vi "CCSelectDICOMitemTags.vi"() -> ()   [LabVIEW 2013, in "ClearCanvasLibrary.lvlib"]
uses:
  ClearCanvasLibrary.lvlib
  main.lvlib
  C:/Users/Simon/SkyDrive/LabView/2013/DM2020/DICOM/ClearCanvasNewBuild/ClearCanvas.Dicom.dll
  ClearCanvasNewBuild/ClearCanvas.Dicom.dll
panel:
  out "Item Symbols":i32[](array[numeric])
  in  "Listbox":i32[](listbox)
  out "error out":errorcluster
  in  "error in (no error)":errorcluster
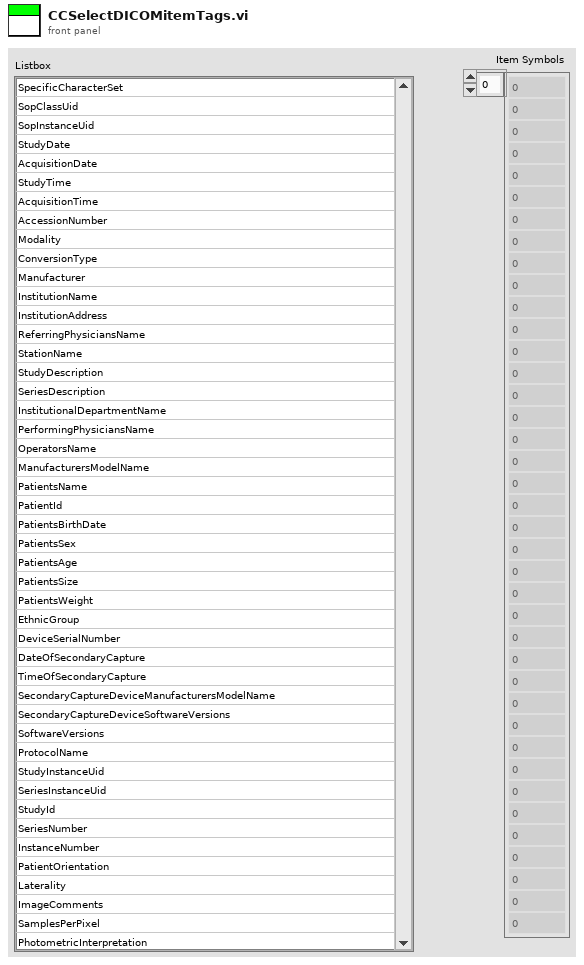
[diagram p1: front panel]
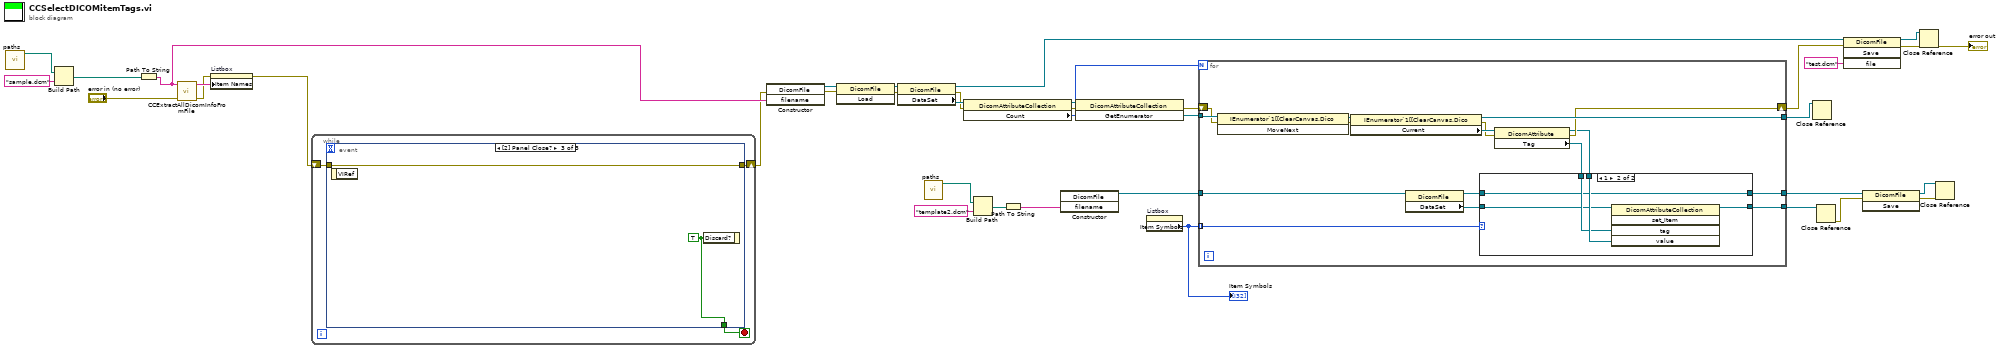
[diagram p0: block diagram]
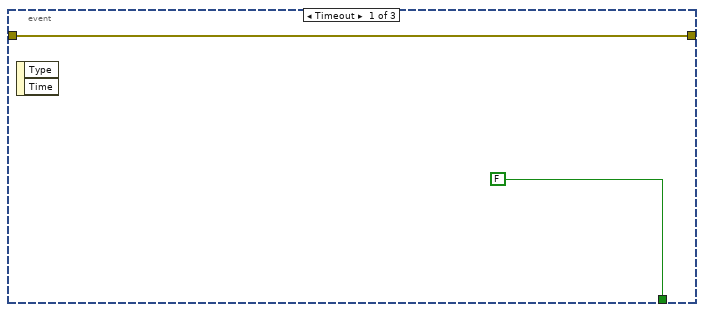
[diagram p3: hidden frame]
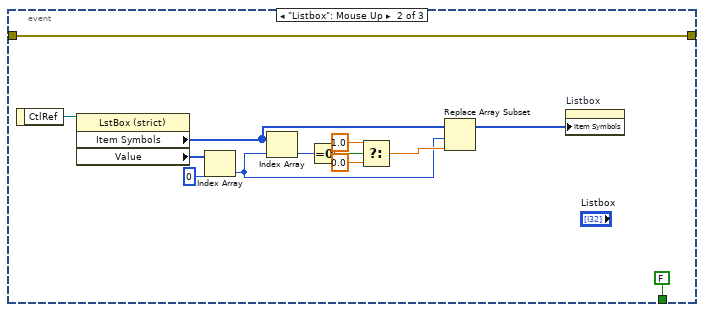
[diagram p4: hidden frame]
diagram:
  n1 = call "paths.vi"() -> ("PubAppData"=w37:path)  [unwired: 8 in, 3 out]
  n2 = Build Path(base path=w37, name or relative path="sample.dcm") -> (appended path=w35:path)
  n3 = Path To String(path=w35) -> (string=w22:string)
  n4 = call "CCExtractAllDicomInfoFromFile.vi"("error in (no error)"="error in (no error)", "filename"=w22) -> ("error out"=w33:errorcluster, "VariableName"=w34:string[])  [unwired: 7 in, 1 out]
  n5 = property on="Listbox" class="LstBox (strict)"(error in=w33, "Item Names"=w34) -> (error out=w17:errorcluster)  [unwired: 1 in, 1 out]
  n6 = while {
    shift-right: [w39] -> w16
    shift-left: w17 -> [w40]
    stop <- w41 stop-if-true
    n7 = event shown="[2] Panel Close?" {
      selector: _ -> [_ _ _]
      dyn-events: _ -> [_ _ _]
      timeout: _ -> [_ _ _]
      tunnel: [FALSE FALSE w58] -> w41
      tunnel: w40 -> [w42 w44 w57]
      tunnel: [w42 w44 w57] -> w39
      event Timeout {
        n8 = event-data() -> ()  [unwired: 1 in, 2 out]
      }
      event "Listbox": Mouse Up {
        n9 = event-data() -> ("CtlRef"=w55:refnum<vi>)  [unwired: 1 in]
        n10 = property class="LstBox (strict)"(reference=w55) -> ("Item Symbols"=w48:i32[], "Value"=w54:i32[])  [unwired: 1 in, 2 out]
        n11 = Index Array(array=w54, index=0) -> (element=w46:i32)
        n12 = Index Array(array=w48, index=w46) -> (element=w52:i32)
        n13 = Equal To 0?(x=w52) -> (x = 0?=w51:bool)
        n14 = Select(t=1.0, s=w51, f=0.0) -> (s? t:f=w47:dbl)
        n15 = Replace Array Subset(array=w48, new element=w47, index=w46) -> (w45:i32[])
        n16 = property on="Listbox" class="LstBox (strict)"("Item Symbols"=w45) -> ()  [unwired: 2 in, 2 out]
      }
      event Panel Close? {
        w58 = TRUE ("Discard?")
        n17 = event-data() -> ()  [unwired: 1 in, 1 out]
        n18 = event-data("Discard?"=w58) -> ()  [unwired: 1 in, 1 out]
      }
    }
  }
  n19 = constructor class="DicomFile"(error in=w16, "filename"=w22) -> (reference out=w21:refnum<k24>, error out=w18:errorcluster)  [unwired: 2 in, 2 out]
  n20 = invoke class="DicomFile" method="Load"(reference=w21, error in=w18) -> (reference out=w20:refnum<k24>, error out=w19:errorcluster)  [unwired: 1 in, 1 out]
  n21 = property class="DicomFile"(reference=w20, error in=w19) -> (reference out=w25:refnum<k24>, error out=w28:errorcluster, "DataSet"=w32:refnum<k24>)
  n22 = call "paths.vi"() -> ("PubAppData"=w15:path)  [unwired: 8 in, 3 out]
  n23 = property class="DicomAttributeCollection"(reference=w32, error in=w28) -> (reference out=w31:refnum<k24>, error out=w27:errorcluster, "Count"=w30:i32)
  n24 = Build Path(base path=w15, name or relative path="template2.dcm") -> (appended path=w13:path)
  n25 = Path To String(path=w13) -> (string=w12:string)
  n26 = constructor class="DicomFile"("filename"=w12) -> (reference out=w11:refnum<k24>)  [unwired: 3 in, 3 out]
  n27 = invoke class="DicomAttributeCollection" method="GetEnumerator"(reference=w31, error in=w27) -> (error out=w26:errorcluster, "GetEnumerator"=w29:refnum<k24>)  [unwired: 1 in, 1 out]
  n28 = property on="Listbox" class="LstBox (strict)"() -> ("Item Symbols"=w10:i32[])  [unwired: 2 in, 2 out]
  "Item Symbols" <- w10
  n29 = for {
    N: w30 -> [_]
    tunnel: w29 -> [w74]
    tunnel: [w72] -> w1
    shift-right: [w67] -> w24
    shift-left: w26 -> [w71]
    tunnel: w11 -> [w60]
    tunnel: [w64] -> w6
    tunnel: w10 -> [w63] mode=indexing
    tunnel: [w59] -> w9
    n30 = invoke class="IEnumerator`1[[ClearCanvas.Dico" method="MoveNext"(reference=w74, error in=w71) -> (reference out=w73:refnum<k24>, error out=w70:errorcluster)  [unwired: 1 in, 1 out]
    n31 = property class="IEnumerator`1[[ClearCanvas.Dico"(reference=w73, error in=w70) -> (reference out=w72:refnum<k24>, error out=w68:errorcluster, "Current"=w69:refnum<k24>)
    n32 = property class="DicomFile"(reference=w60) -> (reference out=w62:refnum<k24>, "DataSet"=w61:refnum<k24>)  [unwired: 1 in, 1 out]
    n33 = property class="DicomAttribute"(reference=w69, error in=w68) -> (reference out=w66:refnum<k24>, error out=w67:errorcluster, "Tag"=w65:refnum<k24>)
    n34 = case shown="1" w63 {
      tunnel: w62 -> [w76 w77]
      tunnel: w66 -> [_ w81]
      tunnel: w65 -> [_ w80]
      tunnel: [w76 w77] -> w59
      tunnel: [w75 w79] -> w64
      tunnel: w61 -> [w75 w78]
      frame 0, Default {
      }
      frame 1 {
        n35 = invoke class="DicomAttributeCollection" method="set_Item"(reference=w78, "tag"=w80, "value"=w81) -> (reference out=w79:refnum<k24>)  [unwired: 2 in, 4 out]
      }
    }
  }
  n36 = Close Reference(reference=w1) -> ()  [unwired: 1 in, 1 out]
  n37 = Close Reference(reference=w6) -> (error out=w5:errorcluster)  [unwired: 1 in]
  n38 = invoke class="DicomFile" method="Save"(reference=w25, error in=w24, "file"="test.dcm") -> (reference out=w3:refnum<k24>, error out=w4:errorcluster)  [unwired: 1 in, 2 out]
  n39 = invoke class="DicomFile" method="Save"(reference=w9, error in=w5) -> (reference out=w7:refnum<k24>, error out=w8:errorcluster)  [unwired: 1 in, 1 out]
  n40 = Close Reference(reference=w3, error in (no error)=w4) -> (error out=→"error out":errorcluster)
  n41 = Close Reference(reference=w7, error in (no error)=w8) -> ()  [unwired: 1 out]
